vi "PXI-Enumerate DIO Ports.vi"(0 "Direction":enum16{"Input", "Output"}(ring), 7 "Must be buffered":bool, 11 "error in (no error)":errorcluster) -> (4 "Ports":tag[](array[tag]), 15 "error out":errorcluster)   [LabVIEW 2020]
uses:
  <resource>/objmgr/daqmx.rc
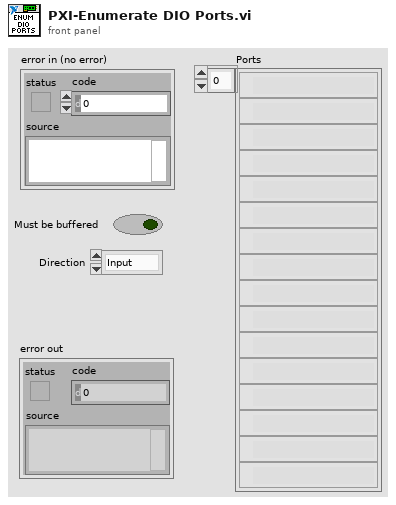
[diagram p1: front panel]
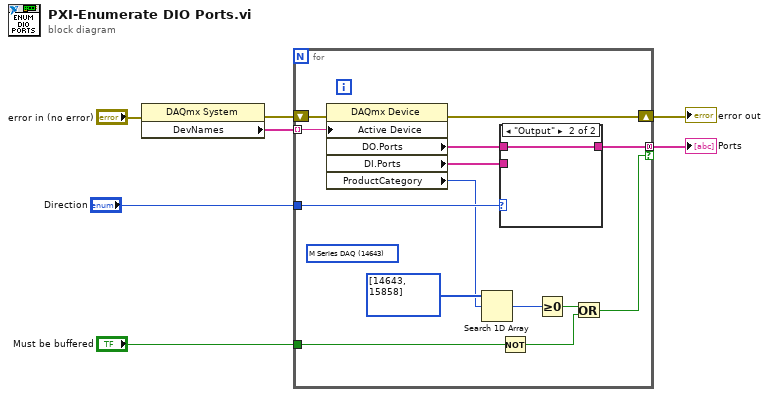
[diagram p0: block diagram]
diagram:
  n1 = property class="DAQmx System"(error in="error in (no error)") -> (error out=w5:errorcluster, "DevNames"=w6:tag[])  [unwired: 1 in, 1 out]
  n2 = for {
    tunnel: w6 -> [w20] mode=indexing
    shift-right: [w21] -> w4
    shift-left: w5 -> [w19]
    tunnel: [w15] -> w2 mode=concatenating if=w8
    tunnel: "Direction" -> [w18]
    tunnel: "Must be buffered" -> [w10]
    (unwired) 14643 items=["M Series DAQ"=14643, "X Series DAQ"=15858, "E Series DAQ"=14642, "S Series DAQ"=14644, "B Series DAQ"=14662, "SC Series DAQ"=14645, "USB DAQ"=14646, "AO Series"=14647, "Digital I/O"=14648, "TIO Series"=14661, "Dynamic Signal Acquisition"=14649, "Switches"=14650, "CompactDAQ Chassis"=14658, "C Series Module"=14659, "SCXI Module"=14660, "SCC Connector Block"=14704, "SCC Module"=14705, "NI ELVIS"=14755, "Network DAQ"=14829, "SC Express"=15886, "Unknown"=12588] ("ProductCategory")
    n3 = property class="DAQmx Device"(error in=w19, "Active Device"=w20) -> (error out=w21:errorcluster, "DO.Ports"=w17:tag[], "DI.Ports"=w16:tag[], "ProductCategory"=w13:i32)  [unwired: 1 in, 1 out]
    n4 = Search 1D Array(1D array=i32[] [14643, 15858], element=w13) -> (index of element=w12:i32)  [unwired: 1 in]
    n5 = case shown="\"Output\"" w18 {
      tunnel: w17 -> [_ w23]
      tunnel: w16 -> [w22 _]
      tunnel: [w22 w23] -> w15
      frame "Input", Default {
      }
      frame "Output" {
      }
    }
    n6 = Not(x=w10) -> (.not. x?=w9:bool)
    n7 = Greater Or Equal To 0?(x=w12) -> (x >= 0?=w11:bool)
    n8 = Or(x=w11, y=w9) -> (x .or. y?=w8:bool)
  }
  "error out" <- w4
  "Ports" <- w2
